vi "Untitled 3.vi"() -> ()   [LabVIEW 2017]
panel:
  in  "message":string="Hello world"
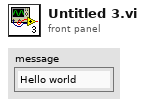
[diagram p1: front panel]
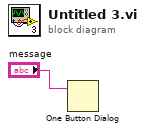
[diagram p0: block diagram]
diagram:
  n1 = One Button Dialog(message="message") -> ()  [unwired: 1 in, 1 out]
